vi "Dark model linear fit.vi"(9 "Frequencies":dbl[](array[numeric]), 10 "Integration Times":dbl[](array[numeric]), 11 "Scans":dbl[][](array[numeric])) -> (1 "Residuals":dbl[][](array[numeric]), 2 "Intercepts":dbl[](array[numeric]), 3 "Slopes":dbl[](array[numeric]))   [LabVIEW 2014, in "AvaSpec.lvlib" / "Dark.lvlib"]
uses:
  Dark.lvlib
  <vilib>/Analysis/NI_AALPro.lvlib
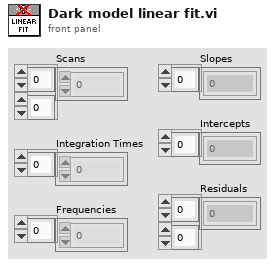
[diagram p1: front panel]
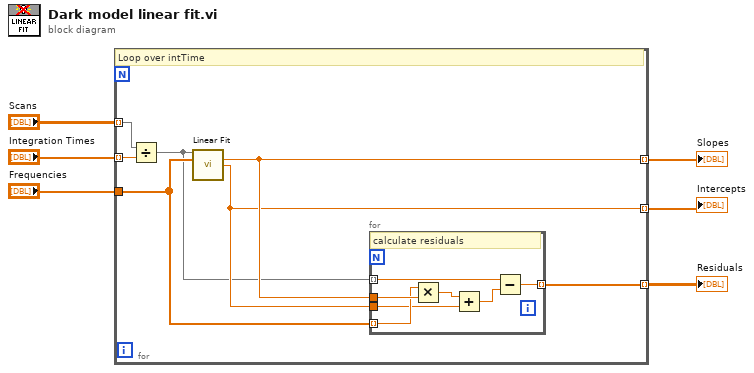
[diagram p0: block diagram]
diagram:
  n1 = for {
    tunnel: "Scans" -> [w10] mode=indexing
    tunnel: "Integration Times" -> [w8] mode=indexing
    tunnel: "Frequencies" -> [w13]
    tunnel: [w12] -> w4 mode=indexing
    tunnel: [w11] -> w5 mode=indexing
    tunnel: [w9] -> w2 mode=indexing
    # "Loop over intTime"
    n2 = Divide(x=w10, y=w8) -> (x/y=w7:dbl[])
    n3 = call <vilib>:"Linear Fit.vi"("Y"=w7, "X"=w13) -> ("slope"=w12:dbl, "intercept"=w11:dbl)  [unwired: 9 in, 3 out]
    n4 = for {
      tunnel: w13 -> [w19] mode=indexing
      tunnel: w12 -> [w20]
      tunnel: w11 -> [w17]
      tunnel: w7 -> [w15] mode=indexing
      tunnel: [w14] -> w9 mode=indexing
      # "calculate residuals"
      n5 = Multiply(x=w19, y=w20) -> (x*y=w18:dbl)
      n6 = Add(x=w18, y=w17) -> (x+y=w16:dbl)
      n7 = Subtract(x=w15, y=w16) -> (x-y=w14:dbl)
    }
  }
  "Intercepts" <- w5
  "Slopes" <- w4
  "Residuals" <- w2
